vi "Chronos TDMS Create Array Dimensions from Index Text.vi"(8 "error in (no error)":errorcluster, 11 "index string":string) -> (0 "error out":errorcluster, 3 "Indecies":i32[](array[numeric]))   [LabVIEW 2021]
uses:
  <vilib>/regexp/Match Regular Expression.xnode
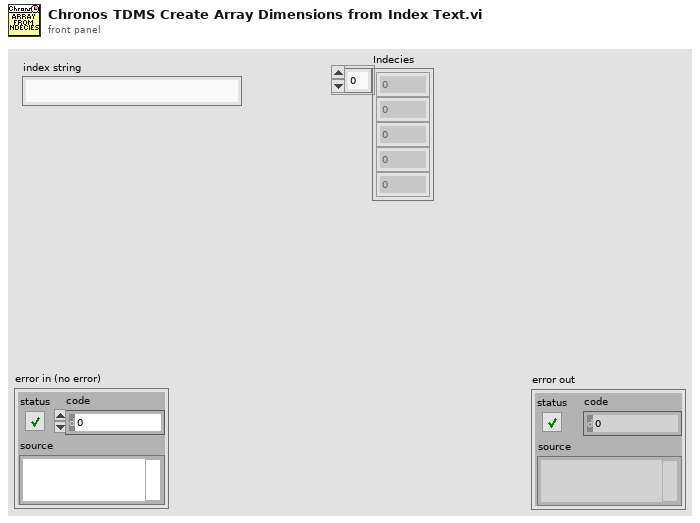
[diagram p1: front panel]
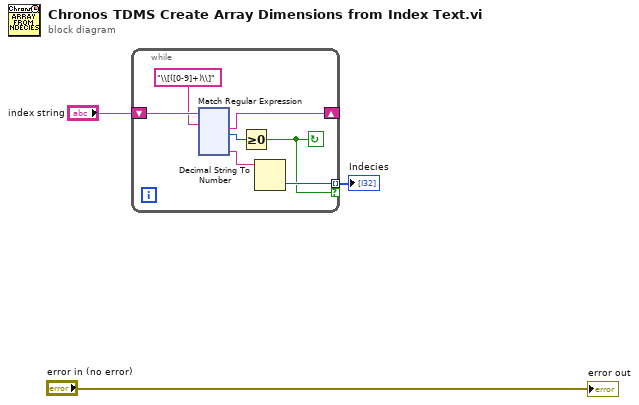
[diagram p0: block diagram]
diagram:
  n1 = while {
    shift-right: [w9] -> _
    shift-left: "index string" -> [w10]
    tunnel: [w6] -> w2 mode=indexing if=w4
    stop <- w4 continue-if-true
    n2 = xnode "Match Regular Expression"("input string"=w10, "regular expression"="\\[([0-9]+)\\]") -> ("after match"=w9:string, "offset past match"=w5:i32, "submatch 1"=w7:string)  [unwired: 4 in, 3 out]
    n3 = Greater Or Equal To 0?(x=w5) -> (x >= 0?=w4:bool)
    n4 = Decimal String To Number(string=w7) -> (number=w6:i32)  [unwired: 2 in, 1 out]
  }
  "Indecies" <- w2
  "error out" <- "error in (no error)"
